vi "MoveMemory.vi"(8 "error in (no error)":errorcluster, 9 "puLen":i32, 10 "lplpBuffer":i32, 11 "Datatype":T1(ring)) -> (0 "error out":errorcluster, 2 "data":string)   [LabVIEW 2015]
doc: "This VI calls the kernel32.dll routine RtlMoveMemory. The RtlMoveMemory routine moves memory either forward or backward, aligned or unaligned, in 4-byte blocks, followed by any remaining bytes.\n\nThis VI copies memory from a location specified by a pointer and its size into a LabVIEW variable. This VI can copy data into an array of words, a FixedFileInfo cluster, or a language code cluster, depending on its configuration."
uses:
  FixedFileInfo_Struct.ctl
  kernel32.dll
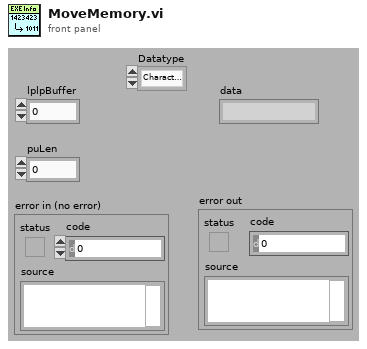
[diagram p1: front panel]
types:
  T1 = enum16{"CharacterArray", "FixedFileInfoCluster", "LanguageCode"}
  T2 = typedef "FixedFileInfo_Struct.ctl" = cluster{"dwSignature":i32, "dwStrucVersionl":i16, "dwStrucVersionh":i16, "dwFileVersionMSl":i16, "dwFileVersionMSh":i16, "dwFileVersionLSl":i16, "dwFileVersionLSh":i16, "dwProductVersionMSl":i16, "dwProductVersionMSh":i16, "dwProductVersionLSl":i16, "dwProductVersionLSh":i16, "dwFileFlagsMask":i32, "dwFileFlags":i32, "dwFileOS":i32, "dwFileType":i32, "dwFileSubtype":i32, "dwFileDateMS":i32, "dwFileDateLS":i32}
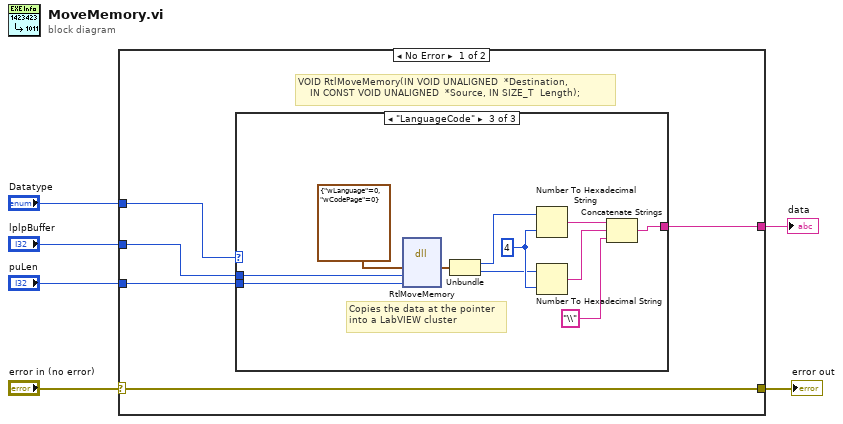
[diagram p0: block diagram]
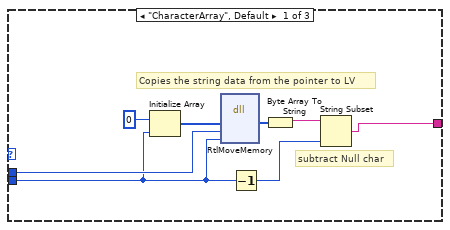
[diagram p2: hidden frame]
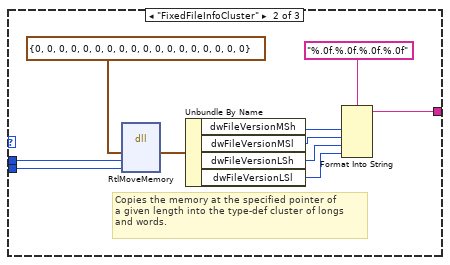
[diagram p3: hidden frame]
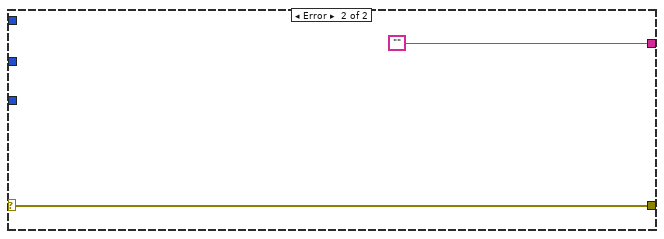
[diagram p4: hidden frame]
diagram:
  n1 = case shown="No Error" "error in (no error)" {
    selector: "error in (no error)" -> [w11 w42]
    tunnel: [w11 w42] -> w5
    tunnel: "lplpBuffer" -> [w10 _]
    tunnel: "puLen" -> [w9 _]
    tunnel: [w8 "" ("string")] -> w2
    tunnel: "Datatype" -> [w7 _]
    frame No Error {
      # "VOID RtlMoveMemory(IN VOID UNALIGNED  *Destination,\n    IN CONST VOID UNALIGNED  *Source, IN SIZE_T  Length);"
      n2 = case shown="\"LanguageCode\"" w7 {
        tunnel: w10 -> [w14 w22 w32]
        tunnel: w9 -> [w12 w21 w31]
        tunnel: [w13 w20 w33] -> w8
        frame "CharacterArray", Default {
          # "Copies the string data from the pointer to LV"
          # "subtract Null char"
          n3 = Initialize Array(u8 0 ("width (-)"), w12) -> (w18:u8[])
          n4 = dll-call lib="kernel32.dll" fn="RtlMoveMemory"("dest"=w18, "Source"=w14, "length"=w12) -> ("dest"=w17:u8[])  [unwired: 6 in, 2 out]
          n5 = Decrement(x=w12) -> (x-1=w15:i32)
          n6 = Byte Array To String(unsigned byte array=w17) -> (string=w16:string)
          n7 = String Subset(string=w16, length (rest)=w15) -> (substring=w13:string)  [unwired: 1 in]
        }
        frame "FixedFileInfoCluster" {
          # "Copies the memory at the specified pointer of\na given length into the type-def cluster of longs\nand words."
          n8 = dll-call lib="kernel32.dll" fn="RtlMoveMemory"("FixedFileInfo Struct"=T2 {"dwSignature"=0, "dwStrucVersionl"=0, "dwStrucVersionh"=0, "dwFileVersionMSl"=0, "dwFileVersionMSh"=0, "dwFileVersionLSl"=0, "dwFileVersionLSh"=0, "dwProductVersionMSl"=0, "dwProductVersionMSh"=0, "dwProductVersionLSl"=0, "dwProductVersionLSh"=0, "dwFileFlagsMask"=0, "dwFileFlags"=0, "dwFileOS"=0, "dwFileType"=0, "dwFileSubtype"=0, "dwFileDateMS"=0, "dwFileDateLS"=0}, "Source"=w22, "length"=w21) -> ("FixedFileInfo Struct"=w28:T2)  [unwired: 6 in, 2 out]
          n9 = Unbundle By Name(w28) -> ("dwFileVersionMSh"=w23:i16, "dwFileVersionMSl"=w25:i16, "dwFileVersionLSh"=w26:i16, "dwFileVersionLSl"=w27:i16)
          n10 = Format Into String(format string="%.0f.%.0f.%.0f.%.0f", w23, w25, w26, w27) -> (resulting string=w20:string)  [unwired: 2 in, 1 out]
        }
        frame "LanguageCode" {
          w40 = i16 4 ("width (-)")
          # "Copies the data at the pointer\ninto a LabVIEW cluster"
          n11 = dll-call lib="kernel32.dll" fn="RtlMoveMemory"(cluster{"wLanguage":i16, "wCodePage":i16} {"wLanguage"=0, "wCodePage"=0}, "Source"=w32, "length"=w31) -> (w37:cluster{"wLanguage":i16, "wCodePage":i16})  [unwired: 6 in, 2 out]
          n12 = Unbundle(w37) -> ("wLanguage"=w38:i16, "wCodePage"=w39:i16)
          n13 = Number To Hexadecimal String(1:w40, 2:w38) -> (0:w35:string)
          n14 = Number To Hexadecimal String(1:w40, 2:w39) -> (0:w34:string)
          n15 = Concatenate Strings(w35, w34, "\\" ("lpSubBlock")) -> (w33:string)
        }
      }
    }
    frame Error {
    }
  }
  "error out" <- w5
  "data" <- w2
